vi "O3 ThermoScientific 49.vi"(8 "error in (no error)":errorcluster) -> (0 "error out":errorcluster={"status"=TRUE, "code"=-1073807338, "source"="VISA Close in O3 ThermoScientific 49.vi"})   [LabVIEW 2013]
doc: "Use this template to build a VI to use as a subVI."
uses:
  <vilib>/Instr/_visa.llb/VISA Configure Serial Port (Instr).vi
  <vilib>/Utility/file.llb/Write To Spreadsheet File (string).vi
panel:
  out "read buffer":string="o3 3353E-2 ppb\r"
  in  "Emulation":bool
  in  "Serial Port Number":refnum<visa-resource-name>="COM3"
  in  "Save to File":bool=TRUE
  in  "file path":path=path "C:/Users/DMA2011/Desktop/o3Conc.txt"
  in  "stop":bool
  out "Waveform Chart":waveform(dbl)(graph)={"t0"=timestamp(3546844894.045 s since 1904-01-01), "dt"=1000.0, "Y"=[33.53]}
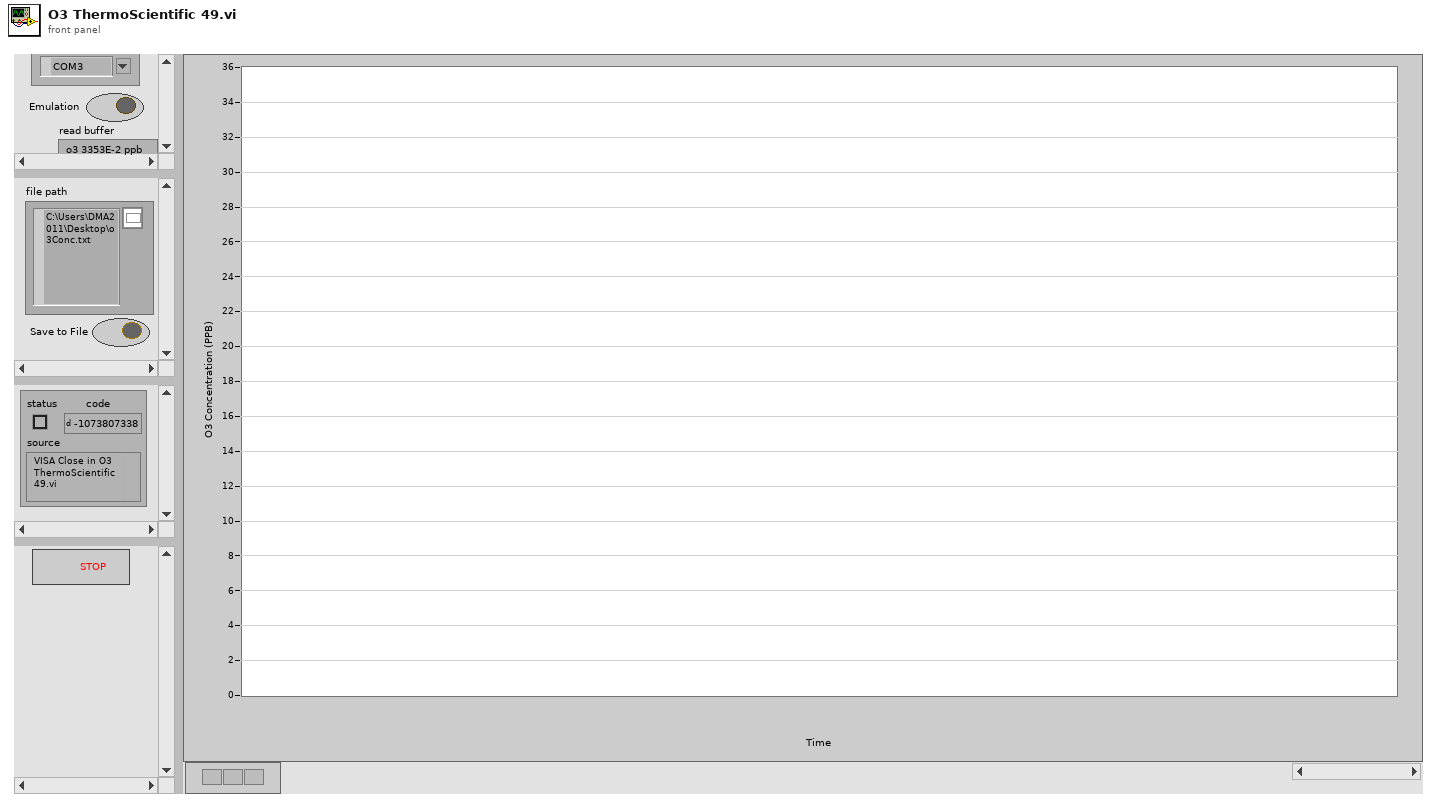
[diagram p1: front panel]
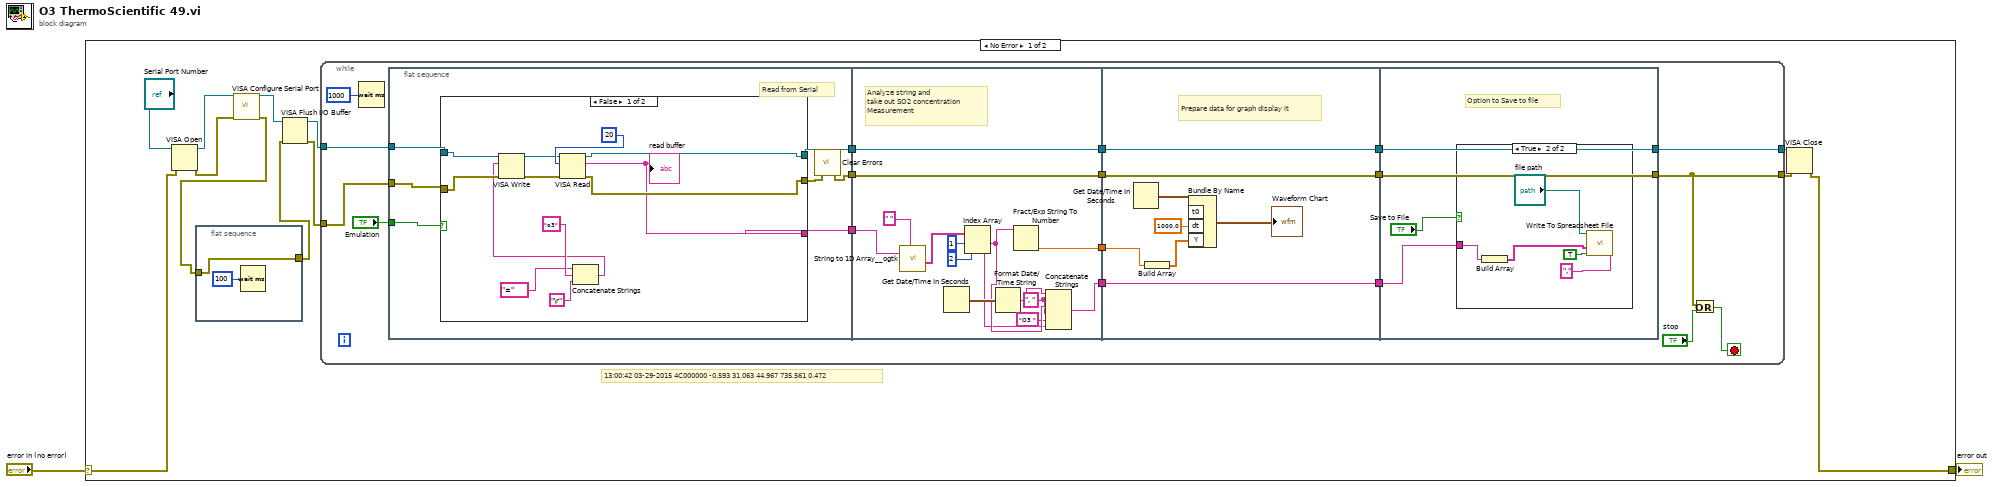
[diagram p0: block diagram]
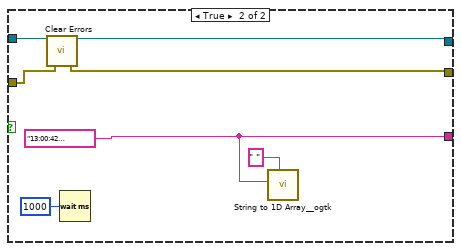
[diagram p2: hidden frame]
diagram:
  n1 = case shown="No Error" "error in (no error)" {
    selector: "error in (no error)" -> [w13 w92]
    tunnel: [w10 w92] -> w1
    frame No Error {
      # "13:00:42 03-29-2015 4C000000 -0.593 31.063 44.967 735.561 0.472"
      n2 = VISA Open(error in (no error)=w13, VISA resource name="Serial Port Number") -> (VISA resource name=w9:refnum<visa-resource-name>, error out=w8:errorcluster)  [unwired: 3 in]
      n3 = flat-sequence {
        tunnel: w7 -> [w15]
        tunnel: [w15] -> w4
        frame #0 {
          n4 = Wait (ms)(milliseconds to wait=u32 100) -> ()  [unwired: 1 out]
        }
      }
      n5 = call-poly "VISA Configure Serial Port"("VISA resource name"=w9, "error in (no error)"=w8) -> ("VISA resource name out"=w6:refnum<visa-resource-name>, "error out"=w7:errorcluster)  [unwired: 12 in]
      n6 = VISA Flush I/O Buffer(VISA resource name=w6, error in (no error)=w4) -> (VISA resource name out=w5:refnum<visa-resource-name>, error out=w3:errorcluster)  [unwired: 1 in]
      n7 = while {
        tunnel: w5 -> [w34]
        tunnel: w3 -> [w28]
        tunnel: [w31] -> w12
        tunnel: [w33] -> w11
        stop <- w30 stop-if-true
        n8 = Wait (ms)(milliseconds to wait=u32 1000) -> ()  [unwired: 1 out]
        n9 = flat-sequence {
          tunnel: w34 -> [w41]
          tunnel: "Emulation" -> [w39]
          tunnel: w28 -> [w37]
          tunnel: [w40] -> w27
          tunnel: [w35] -> w26
          tunnel: [w38] -> w25
          tunnel: w27 -> [w74]
          tunnel: w26 -> [w68]
          tunnel: w25 -> [w73]
          tunnel: [w74] -> w24
          tunnel: [w72] -> w23
          tunnel: [w68] -> w20
          tunnel: [w64] -> w18
          tunnel: w24 -> [w82]
          tunnel: w23 -> [w81]
          tunnel: [w82] -> w22
          tunnel: [w76] -> w21
          tunnel: w20 -> [w76]
          tunnel: [w75] -> w19
          tunnel: w18 -> [w75]
          tunnel: [w85] -> w31
          tunnel: [w86] -> w33
          tunnel: w22 -> [w86]
          tunnel: w21 -> [w85]
          tunnel: w19 -> [w83]
          frame #0 {
            # "Read from Serial"
            n10 = case shown="False" w39 {
              tunnel: w41 -> [w52 w59]
              tunnel: [w47 w59] -> w40
              tunnel: [w42 w54] -> w38
              tunnel: [w48 w56] -> w36
              tunnel: w37 -> [w51 w57]
              frame False {
                n11 = Concatenate Strings("±" ("write buffer"), "o3" ("write buffer"), "\r") -> (w44:string)
                n12 = VISA Write(VISA resource name=w52, write buffer=w44, error in (no error)=w51) -> (VISA resource name out=w50:refnum<visa-resource-name>, error out=w49:errorcluster)  [unwired: 1 out]
                n13 = VISA Read(VISA resource name=w50, byte count=u32 20, error in (no error)=w49) -> (VISA resource name out=w47:refnum<visa-resource-name>, read buffer=w42:string, error out=w48:errorcluster)  [unwired: 1 out]
                "read buffer" <- w42
              }
              frame True {
                w54 = "13:00:42 03-29-2015 4C000000 -0.593 31.063 44.967 735.561 0.472"
                n14 = call <vilib>:"Clear Errors.vi"("error in (no error)"=w57) -> ("error out"=w56:errorcluster)  [unwired: 6 in]
                n15 = Wait (ms)(milliseconds to wait=u32 1000) -> ()  [unwired: 1 out]
                n16 = call <userlib>:"String to 1D Array__ogtk.vi"("delimiter (Tab)"=" ", "string"=w54) -> ()  [unwired: 9 in, 1 out]
              }
            }
            n17 = call <vilib>:"Clear Errors.vi"("error in (no error)"=w36) -> ("error out"=w35:errorcluster)  [unwired: 6 in]
          }
          frame #1 {
            w62 = ", " ("string")
            # "Analyze string and\ntake out SO2 concentration\nMeasurement"
            n18 = call <userlib>:"String to 1D Array__ogtk.vi"("delimiter (Tab)"=" ", "string"=w73) -> ("Array of Strings"=w70:string[])  [unwired: 9 in]
            n19 = Get Date/Time In Seconds() -> (seconds since 1Jan1904=w66:timestamp)
            n20 = Index Array(array=w70, index #1=1 ("index"), index #2=2 ("index")) -> (element #1=w65:string, element #2=w61:string)
            n21 = Format Date/Time String(seconds (now)=w66) -> (date/time string=w67:string)  [unwired: 2 in]
            n22 = Fract/Exp String To Number(string=w65) -> (number=w72:dbl)  [unwired: 3 in, 1 out]
            n23 = Concatenate Strings(w67, w62, w65, w62, "O3 " ("string"), w61) -> (w64:string)
          }
          frame #2 {
            # "Prepare data for graph display it"
            n24 = Get Date/Time In Seconds() -> (seconds since 1Jan1904=w80:timestamp)
            n25 = Build Array(w81) -> (w78:dbl[])
            n26 = Bundle By Name("t0"=w80, "dt"=1000.0, "Y"=w78) -> (→"Waveform Chart":waveform(dbl))  [unwired: 1 in]
          }
          frame #3 {
            # "Option to Save to file"
            n27 = case shown="True" "Save to File" {
              tunnel: w83 -> [_ w88]
              frame False {
              }
              frame True {
                n28 = Build Array(w88) -> (w87:string[])
                n29 = call-poly <vilib>:"Write To Spreadsheet File.vi"("delimiter (\\t)"="," ("delimiter (\\t)"), "append to file? (new file:F)"=TRUE, "1D data"=w87, "file path (dialog if empty)"="file path") -> ()  [unwired: 4 in, 1 out]
              }
            }
          }
        }
        n30 = Or(x=w31, y="stop") -> (x .or. y?=w30:bool)
      }
      n31 = VISA Close(VISA resource name=w11, error in (no error)=w12) -> (error out=w10:errorcluster)
    }
    frame Error {
    }
  }
  "error out" <- w1
